vi "Start Queue.vi"(6 "Refs":refnum<class "Refs.lvclass">, 7 "Actor in":refnum<class "Actor.lvclass">, 9 "Actor Ref":refnum<vi>, 10 "Spawn":refnum<class "Spawn.lvclass">) -> (0 "Error out":errorcluster, 5 "Actor out":refnum<class "Actor.lvclass">)   [LabVIEW 2025, in "jettl.lvlib" / "Transport.lvlib" / "Queue.lvlib"]
uses:
  Queue.lvlib
  Refs/Refs.lvclass
  Actor/Actor.lvclass
  Spawn/Spawn/Spawn.lvclass
  Queue Transport/Queue Transport.lvclass
  C:/git/jettl/src/jettl/jettl/Transport/Queue/Queue Transport/Queue Transport.lvclass
  C:/git/jettl/src/jettl/jettl/Transport/Transport/Transport.lvclass
  jettl.lvlib
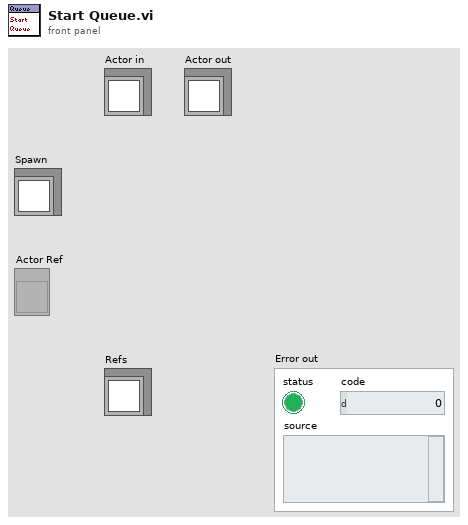
[diagram p1: front panel]
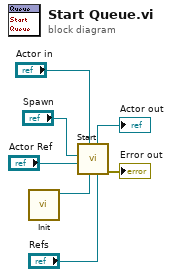
[diagram p0: block diagram]
diagram:
  n1 = call "Init.vi"() -> ("Queue Transport out"=w1:refnum<class "Queue Transport.lvclass">)  [unwired: 11 in]
  n2 = call "Start.vi"("Refs"="Refs", "Transport"=w1, "Actor in"="Actor in", "Actor Ref"="Actor Ref", "Spawn"="Spawn") -> ("Error out"=→"Error out":errorcluster, "Actor out"=→"Actor out":refnum<class "Actor.lvclass">)  [unwired: 5 in]
